vi "Validate.vi"(6 "Length":u8, 8 "error in":errorcluster, 9 "Sub-Index":u8 format="%02x", 10 "Index":u16 format="%04x", 11 "Obj Dict":refnum<class "Object Dictionary.lvclass">) -> (0 "error out":errorcluster, 1 "Valid?":bool, 2 "Sub Obj":refnum<class "Sub Object.lvclass">)   [LabVIEW 2020, in "CANopen.lvlib" / "PDO Mapping.lvclass"]
uses:
  PDO Mapping.lvclass
  PDO Mapping.lvclass/PDO Mapping.ctl
  Object Dictionary/Object Dictionary.lvclass
  Sub Object/Sub Object.lvclass
  CANopen.lvlib
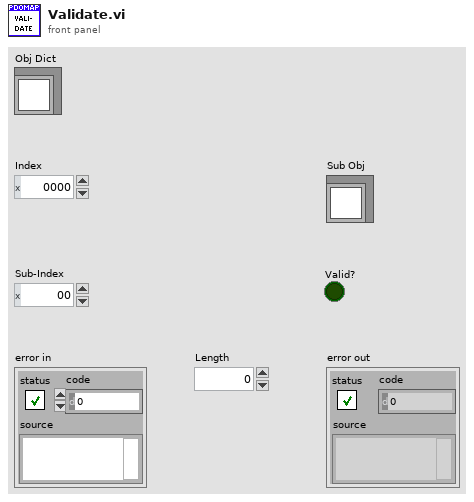
[diagram p1: front panel]
types:
  T1 = typedef "CANopen.lvlib/Data Type.ctl" = u16
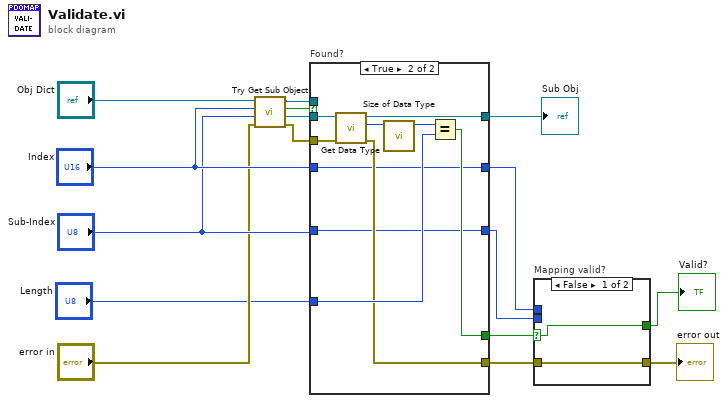
[diagram p0: block diagram]
diagram:
  n1 = call "Try Get Sub Object.vi"("error in"="error in", "Sub Index"="Sub-Index", "Index"="Index", "Object Dictionary in"="Obj Dict") -> ("error out"=w10:errorcluster, "Sub Object"=w2:refnum<class "Sub Object.lvclass">, "Success"=w1:bool, "Object Dictionary out"=w11:refnum<class "Object Dictionary.lvclass">)  [unwired: 4 in]
  n2 = case "Found?" shown="True" w1 {
    selector: w1 -> [w17 _]
    tunnel: [w18 w25] -> w9
    tunnel: "Index" -> [w20 w24]
    tunnel: "Sub-Index" -> [w19 w23]
    tunnel: "Length" -> [_ w27]
    tunnel: w11 -> [_ _]
    tunnel: w2 -> [_ w30]
    tunnel: w10 -> [w18 w29]
    tunnel: [w17 w26] -> w7
    tunnel: [w20 w24] -> w6
    tunnel: [w19 w23] -> w5
    tunnel: [_ w22] -> w3
    frame False {
    }
    frame True {
      n3 = call "Get Data Type.vi"("error in (no error)"=w29, "Sub Object in"=w30) -> ("error out"=w25:errorcluster, "Data Type"=w28:T1, "Sub Object out"=w22:refnum<class "Sub Object.lvclass">)  [unwired: 7 in]
      n4 = call "Size of Data Type.vi"("Data Type"=w28) -> ("Size"=w21:u8)  [unwired: 10 in]
      n5 = Equal?(x=w21, y=w27) -> (x = y?=w26:bool)
    }
  }
  "Sub Obj" <- w3
  n6 = case "Mapping valid?" shown="False" w7 {
    selector: w7 -> [w31 w33]
    tunnel: w9 -> [w32 w34]
    tunnel: [w32 w34] -> w8
    tunnel: w6 -> [_ _]
    tunnel: w5 -> [_ _]
    tunnel: [w31 w33] -> w4
    frame False {
    }
    frame True {
    }
  }
  "error out" <- w8
  "Valid?" <- w4
